vi "update.file.vi"(8 "error in (no error)":errorcluster, 11 "ComicVine_manager in":refnum<class "ComicVine_manager.lvclass">) -> (0 "error out":errorcluster, 3 "ComicVine_manager out":refnum<class "ComicVine_manager.lvclass">)   [LabVIEW 2024, in "ComicVine_manager.lvclass"]
uses:
  ComicVine_manager.lvclass
  ComicVine_manager.lvclass/ComicVine_manager.ctl
  <vilib>/addons/_JKI.lib/Serialization/JSON/JKI JSON Serialization.lvlib
  <userlib>/_OpenG.lib/file/file.llb/openg_file.lvlib
  <userlib>/_OpenG.lib/file/file.llb/Strip Path Extension - String__ogtk.vi
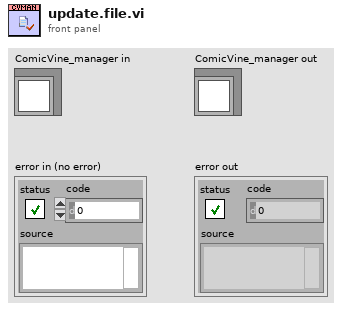
[diagram p1: front panel]
types:
  T1 = typedef "volume.type--enum.ctl" = enum16{"Ongoing", "Limited Series", "Annual", "One Shot", "Reprint/Document"}
  T2 = typedef "local_volume.ctl" = cluster{"id":i32, "name":string, "sortable_name":string, "aliases":string[], "description":string, "site_detail_url":string, "count_of_issues":i32, "start_year":i32, "publisher_id":i32, "issue_ids":i32[], "date_last_updated":timestamp, "volume":i32, "cv_id":string, "volume type":T1}
  T3 = typedef "local_issue.ctl" = cluster{"cover_date":timestamp, "id":i32, "cv_id":string, "name":string, "sortable_name":string, "issue_number":string, "deck":string, "description":string, "volume":T4, "store_date":timestamp, "date_last_updated":timestamp, "site_detail_url":string, "cover_url":string, "associated_images":T5[], "characters":T4[], "concepts":T4[], "creators":T6[], "storyArcs":T4[], "teams":T4[]}
  T4 = typedef "comicvine_issue.generic_credit.ctl" = cluster{"id":i32, "name":string}
  T5 = typedef "comicvine_issue.associated_image.ctl" = cluster{"original_url":string, "id":i32}
  T6 = typedef "comicvine_issue.person_credit.ctl" = cluster{"id":i32, "name":string, "role":string}
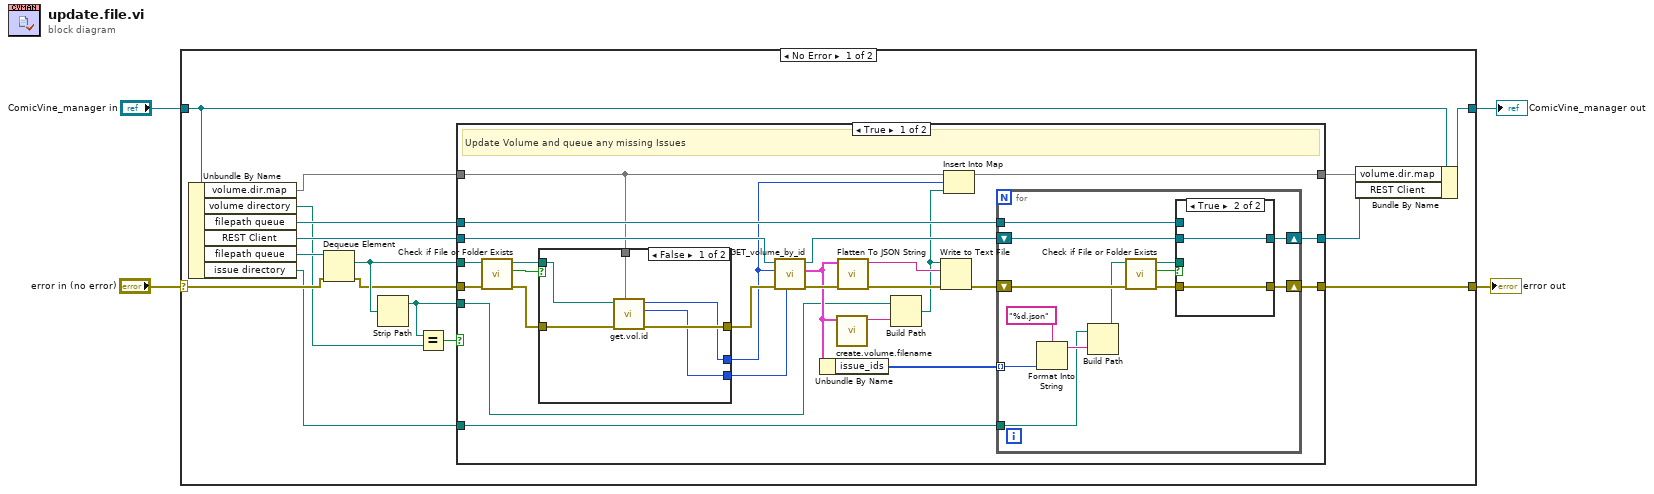
[diagram p0: block diagram]
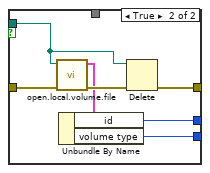
[diagram p2: hidden frame]
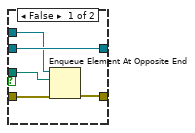
[diagram p3: hidden frame]
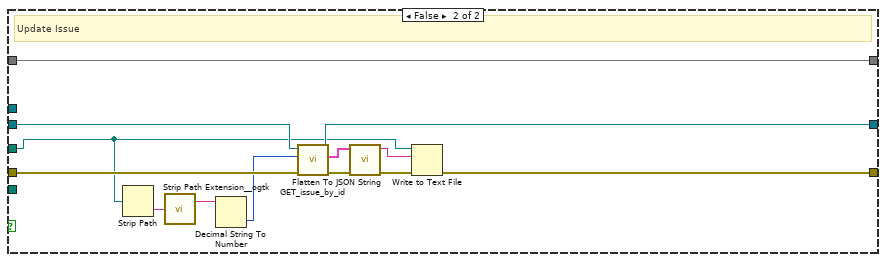
[diagram p4: hidden frame]
diagram:
  n1 = case shown="No Error" "error in (no error)" {
    selector: "error in (no error)" -> [w19 w93]
    tunnel: [w16 w93] -> w3
    tunnel: [w13 w92] -> w1
    tunnel: "ComicVine_manager in" -> [w15 w92]
    frame No Error {
      n2 = Unbundle By Name(w15) -> ("volume.dir.map"=w7:map{i32, path}, "volume directory"=w11:path, "filepath queue"=w12:refnum<queue>, "REST Client"=w18:refnum<class "REST Client.lvclass">, "filepath queue"=w20:refnum<queue>, "issue directory"=w5:path)
      n3 = Dequeue Element(queue=w20, error in (no error)=w19) -> (element=w17:path, error out=w8:errorcluster)  [unwired: 1 in, 2 out]
      n4 = Strip Path(path=w17) -> (stripped path=w10:path)  [unwired: 1 out]
      n5 = Equal?(x=w10, y=w11) -> (x = y?=w9:bool)
      n6 = case shown="True" w9 {
        tunnel: w18 -> [w45 w91]
        tunnel: w8 -> [w33 w90]
        tunnel: w17 -> [w32 w80]
        tunnel: w10 -> [w31 _]
        tunnel: [w35 w85] -> w16
        tunnel: [w38 w84] -> w14
        tunnel: w12 -> [w34 _]
        tunnel: w7 -> [w25 w83]
        tunnel: [w22 w83] -> w6
        tunnel: w5 -> [w21 _]
        frame True {
          # "Update Volume and queue any missing Issues"
          n7 = call <vilib>:"Check if File or Folder Exists.vi"("error in (no error)"=w33, "path"=w32) -> ("error out"=w27:errorcluster, "file or folder exists?"=w28:bool, "dup path"=w30:path)  [unwired: 7 in]
          n8 = case shown="False" w28 {
            tunnel: [w46 w56] -> w23
            tunnel: w30 -> [w48 w55]
            tunnel: [w47 w54] -> w29
            tunnel: w27 -> [w50 w53]
            tunnel: [w51 w52] -> w26
            tunnel: w25 -> [w49 _]
            frame False {
              n9 = call "get.vol.id.vi"("map in"=w49, "error in (no error)"=w50, "Path"=w48) -> ("error out"=w51:errorcluster, "volume type"=w47:T1, "id"=w46:i32)  [unwired: 6 in]
            }
            frame True {
              n10 = call "open.local.volume.file.vi"("error in (no error)"=w53, "volume json"=w55) -> ("error out"=w58:errorcluster, "volume"=w57:T2)  [unwired: 8 in]
              n11 = Unbundle By Name(w57) -> ("id"=w56:i32, "volume type"=w54:T1)
              n12 = Delete(path (use dialog)=w55, error in=w58) -> (error out=w52:errorcluster)  [unwired: 3 in, 2 out]
            }
          }
          n13 = call "GET_volume_by_id.vi"("volume type"=w29, "error in (no error)"=w26, "volume id"=w23, "REST Client in"=w45) -> ("error out"=w43:errorcluster, "local volume"=w40:T2, "REST Client out"=w39:refnum<class "REST Client.lvclass">)  [unwired: 5 in]
          n14 = Unbundle By Name(w40) -> ("issue_ids"=w37:i32[])
          n15 = call "create.volume.filename.vi"("volume"=w40) -> ("json filename"=w44:string)  [unwired: 10 in]
          n16 = call <vilib>:"Flatten To JSON String.vi"("error in (no error)"=w43, "Variant"=w40) -> ("error out"=w41:errorcluster, "JSON String"=w42:string)  [unwired: 8 in]
          n17 = Build Path(base path=w31, name or relative path=w44) -> (appended path=w24:path)
          n18 = Write to Text File(file (use dialog)=w24, text=w42, error in=w41) -> (error out=w36:errorcluster)  [unwired: 1 in, 2 out]
          n19 = Insert Into Map(map in=w25, key=w23, value=w24) -> (map out=w22:map{i32, path})  [unwired: 2 out]
          n20 = for {
            shift-right: [w61] -> w38
            shift-left: w39 -> [w62]
            tunnel: w37 -> [w70] mode=indexing
            tunnel: w21 -> [w68]
            shift-right: [w63] -> w35
            shift-left: w36 -> [w67]
            tunnel: w34 -> [w60]
            n21 = Format Into String(format string="%d.json", w70) -> (resulting string=w69:string)  [unwired: 2 in, 1 out]
            n22 = Build Path(base path=w68, name or relative path=w69) -> (appended path=w66:path)
            n23 = call <vilib>:"Check if File or Folder Exists.vi"("error in (no error)"=w67, "path"=w66) -> ("error out"=w64:errorcluster, "file or folder exists?"=w65:bool, "dup path"=w59:path)  [unwired: 7 in]
            n24 = case shown="True" w65 {
              tunnel: w64 -> [w75 w78]
              tunnel: [w72 w78] -> w63
              tunnel: w62 -> [w76 w77]
              tunnel: [w76 w77] -> w61
              tunnel: w60 -> [w74 _]
              tunnel: w59 -> [w73 _]
              frame False {
                n25 = Enqueue Element At Opposite End(queue=w74, element=w73, error in (no error)=w75) -> (error out=w72:errorcluster)  [unwired: 1 in, 2 out]
              }
              frame True {
              }
            }
          }
        }
        frame False {
          # "Update Issue"
          n26 = Strip Path(path=w80) -> (name=w82:string)  [unwired: 1 out]
          n27 = call-poly <userlib>:"Strip Path Extension__ogtk.vi"("path"=w82) -> ("root"=w81:string)  [unwired: 1 out]
          n28 = Decimal String To Number(string=w81) -> (number=w79:i32)  [unwired: 2 in, 1 out]
          n29 = call "GET_issue_by_id.vi"("error in (no error)"=w90, "issue id"=w79, "REST Client in"=w91) -> ("error out"=w88:errorcluster, "local_issue"=w89:T3, "REST Client out"=w84:refnum<class "REST Client.lvclass">)  [unwired: 6 in]
          n30 = call <vilib>:"Flatten To JSON String.vi"("error in (no error)"=w88, "Variant"=w89) -> ("error out"=w87:errorcluster, "JSON String"=w86:string)  [unwired: 8 in]
          n31 = Write to Text File(file (use dialog)=w80, text=w86, error in=w87) -> (error out=w85:errorcluster)  [unwired: 1 in, 2 out]
        }
      }
      n32 = Bundle By Name(cluster=w15, "volume.dir.map"=w6, "REST Client"=w14) -> (w13:refnum<class "ComicVine_manager.lvclass">)
    }
    frame Error {
    }
  }
  "error out" <- w3
  "ComicVine_manager out" <- w1
